vi "Set Rate (Percent).vi"(8 "error in (no error)":errorcluster, 10 "Percent":dbl, 11 "Elevator in":refnum<class "Elevator.lvclass">) -> (0 "error out":errorcluster, 3 "Elevator out":refnum<class "Elevator.lvclass">)   [LabVIEW 2014, in "Elevator.lvlib" / "Elevator.lvclass"]
uses:
  Elevator.lvclass
  Elevator.lvclass/Elevator.ctl
  Motor with Encoders/Motors with Encoders Messages/Set Rate (Percent) Msg/Set Rate (Percent) Msg.lvclass/Set Rate (Percent) Msg.ctl
  <vilib>/ActorFramework/Message Enqueuer/Message Enqueuer.lvclass/Message Enqueuer.ctl
  <vilib>/ActorFramework/Message Enqueuer/Enqueue.vi
  <vilib>/ActorFramework/Message Priority Queue/Priority Enqueue.vi
  Motor with Encoders/Motors with Encoders Messages/Set Rate (Percent) Msg/Set Rate (Percent) Msg.lvclass
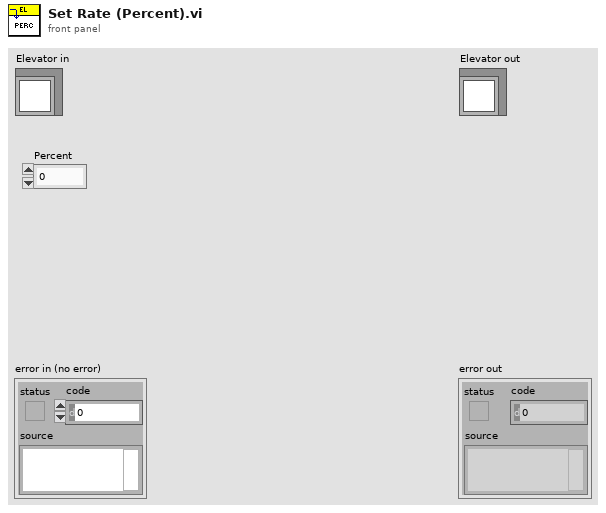
[diagram p1: front panel]
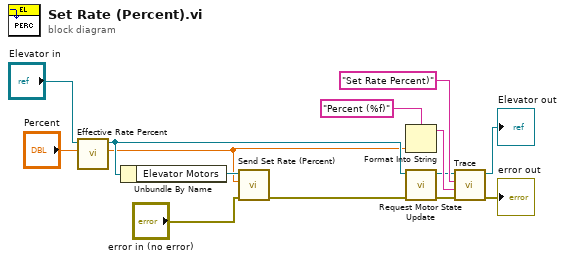
[diagram p0: block diagram]
diagram:
  n1 = call-dynamic "Effective Rate Percent.vi"("Set Rate (Percent) in"="Percent", "Elevator in"="Elevator in") -> ("Set Rate (Percent) out"=w1:dbl, "Elevator out"=w3:refnum<class "Elevator.lvclass">)  [unwired: 7 in, 1 out]
  n2 = Unbundle By Name(w3) -> ("Elevator Motors"=w11:refnum<class "Message Enqueuer.lvclass">)
  n3 = call "Send Set Rate (Percent).vi"("error in (no error)"="error in (no error)", "Rate (Percentage)"=w1, "Message Enqueuer"=w11) -> ("error out"=w6:errorcluster)  [unwired: 7 in, 1 out]
  n4 = Format Into String(format string="Percent (%f)", w1) -> (resulting string=w8:string)  [unwired: 2 in, 1 out]
  n5 = call-dynamic "Request Motor State Update.vi"("error in (no error)"=w6, "Elevator in"=w3) -> ("error out"=w5:errorcluster, "Elevator out"=w7:refnum<class "Elevator.lvclass">)  [unwired: 8 in]
  n6 = call-dynamic "Trace.vi"("error in (no error)"=w5, "System Message"=w8, "System Action"="Set Rate Percent)", "System Actor in"=w7) -> ("error out"=→"error out":errorcluster, "System Actor out"=→"Elevator out":refnum<class "Elevator.lvclass">)  [unwired: 6 in]
